vi "To_More_Generic.vi"(0 "Reference":refnum<vi>[](array[refnum]), 2 "Target _Class":refnum<vi>) -> (4 "Generic_Class reference":refnum<vi>[](array[refnum]))   [LabVIEW 2023]
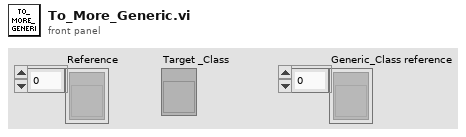
[diagram p1: front panel]
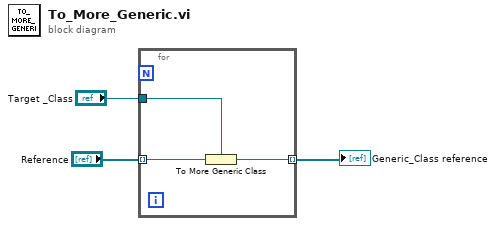
[diagram p0: block diagram]
diagram:
  n1 = for {
    tunnel: "Target _Class" -> [w6]
    tunnel: "Reference" -> [w5] mode=indexing
    tunnel: [w4] -> w1 mode=indexing
    n2 = To More Generic Class(target class=w6, reference=w5) -> (generic class reference=w4:refnum<vi>)
  }
  "Generic_Class reference" <- w1
